vi "test sve.vi"() -> ()   [LabVIEW 2015]
uses:
  <vilib>/Utility/Variable/NI_VariableUtilities.lvlib
panel:
  in  "stop":bool
  in  "obrotowa":dbl
  out "postepowa":dbl
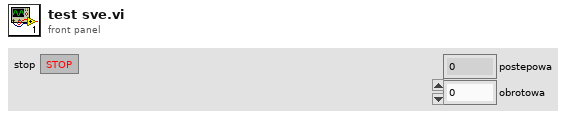
[diagram p1: front panel]
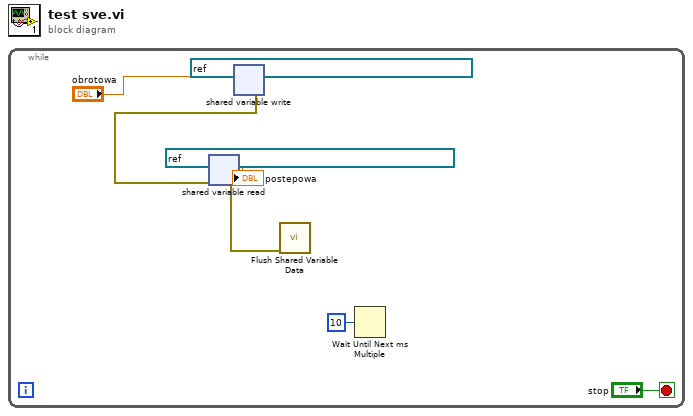
[diagram p0: block diagram]
diagram:
  n1 = while {
    stop <- "stop" stop-if-true
    n2 = shared-variable-write(refnum<k21> "ni.var.psp://lenovo-pc/wspoldzielone/obrotowa" ("shared variable refnum in"), "obrotowa") -> (w4:errorcluster)  [unwired: 1 in, 1 out]
    n3 = shared-variable-read(refnum<k21> "ni.var.psp://lenovo-pc/wspoldzielone/postepowa" ("shared variable refnum in"), w4) -> (w3:errorcluster, →"postepowa":dbl)  [unwired: 1 out]
    n4 = call <vilib>:"Flush Shared Variable Data.vi"("error in (no error)"=w3) -> ()  [unwired: 10 in, 1 out]
    n5 = Wait Until Next ms Multiple(millisecond multiple=u32 10) -> ()  [unwired: 1 out]
  }
